vi "tcs_issueCommand_injectError.vi"(8 "error in (no error)":errorcluster, 11 "command_injectError_Ctl":T1) -> (0 "error out":errorcluster, 2 "function return":i32, 3 "command_injectError_Ctl out":T1)   [LabVIEW 2016, in "SALLV_tcs.lvlib"]
doc: "int tcs_shm_issueCommand_injectErrorLV(tcs_command_injectErrorLV *command_injectError_Ctl );"
uses:
  SALLV_tcs.lvlib
  DataTypes/command_injectError.ctl
  SALLV_tcs.so
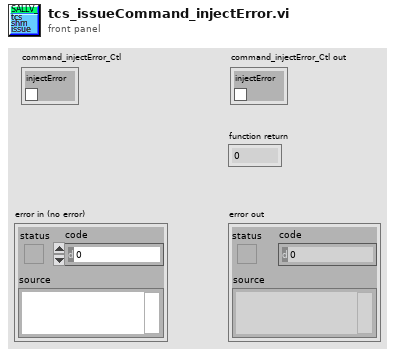
[diagram p1: front panel]
types:
  T1 = typedef "SALLV_tcs.lvlib/command_injectError.ctl" = cluster{"injectError":bool}
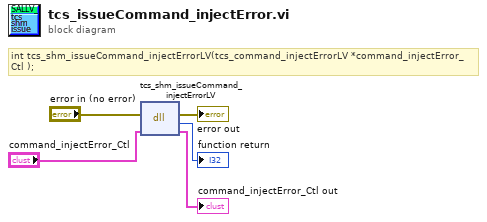
[diagram p0: block diagram]
diagram:
  # "int tcs_shm_issueCommand_injectErrorLV(tcs_command_injectErrorLV *command_injectError_Ctl );"
  n1 = dll-call lib="home/saluser/ct_tcs/ts_sallv_tcs/SALLV_tcs.*" fn="tcs_shm_issueCommand_injectErrorLV"(error in="error in (no error)", "command_injectError_Ctl"="command_injectError_Ctl") -> (error out=→"error out":errorcluster, →"function return":i32, "command_injectError_Ctl"=→"command_injectError_Ctl out":T1)  [unwired: 2 in, 1 out]
